vi "Button Event.vi"(9 "Buttons":bool[](array[boolean])) -> (0 "Button Release":bool[](array[boolean]), 1 "Button Press":bool[](array[boolean]), 3 "Buttons State":bool[](array[boolean]))   [LabVIEW 2014]
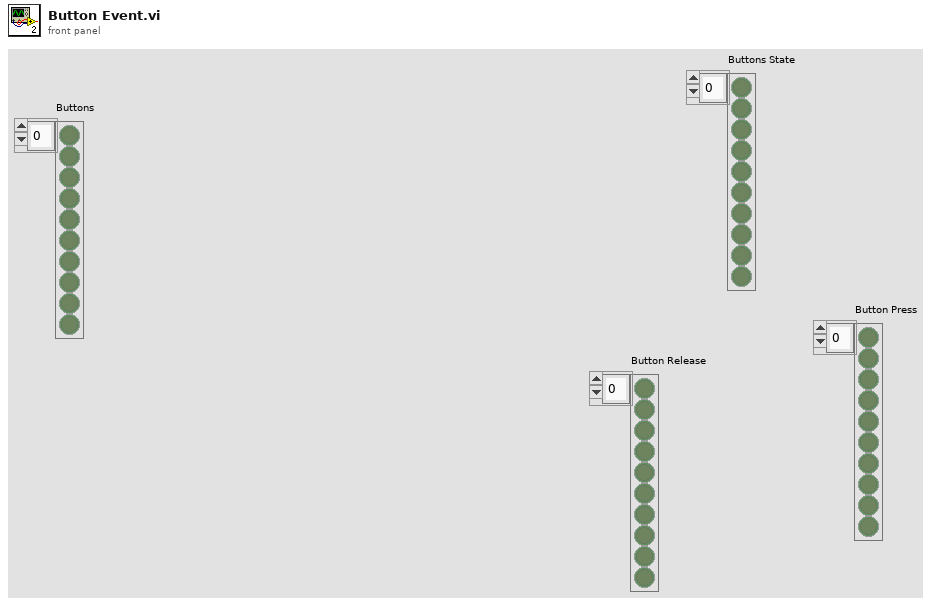
[diagram p1: front panel]
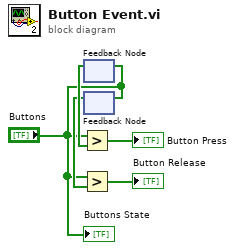
[diagram p0: block diagram]
diagram:
  n1 = feedback-in #1("Buttons") -> ()
  n2 = feedback #1() -> (w4:bool[])  [unwired: 1 in]
  n3 = Greater?(x="Buttons", y=w4) -> (0:→"Button Press":bool[])
  n4 = feedback #2() -> (w2:bool[])  [unwired: 1 in]
  n5 = Greater?(x="Buttons", y=w2) -> (0:→"Button Release":bool[])
  n6 = feedback-in #2("Buttons") -> ()
  "Buttons State" <- "Buttons"
